vi "Run.vi"(8 "error in (no error)":errorcluster, 11 "Opctics in":refnum<class "Optics.lvclass">) -> (0 "error out":errorcluster, 3 "Optics out":refnum<class "Optics.lvclass">)   [LabVIEW 2018, in "Optics.lvclass"]
uses:
  Optics.lvclass
  C:/Users/observer/Desktop/Sparc4GUI/SPARC4_GUI/Device/Device.lvclass
  Optics.lvclass/Optics.ctl
  Device.lvclass/Device.ctl
  Device.lvclass
  StateMachine/State Machine.lvclass
panel:
  out "on target 2":bool
  out "moving2 2":bool
  out "moving1 2":bool
  out "moving3 2":bool
  out "moving3":bool
  out "moving2":bool
  out "moving1":bool
  out "on target":bool
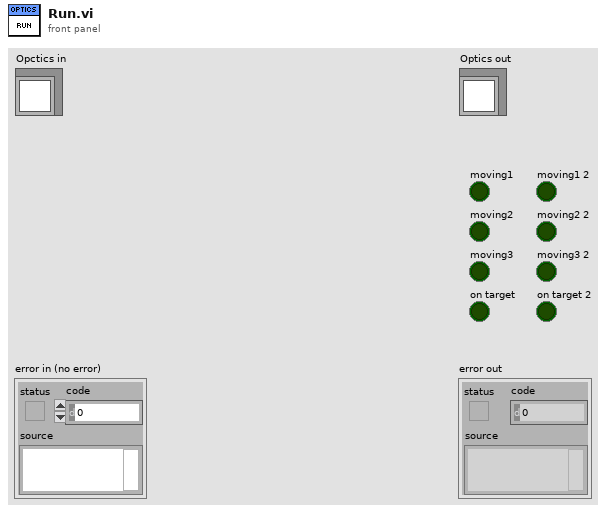
[diagram p1: front panel]
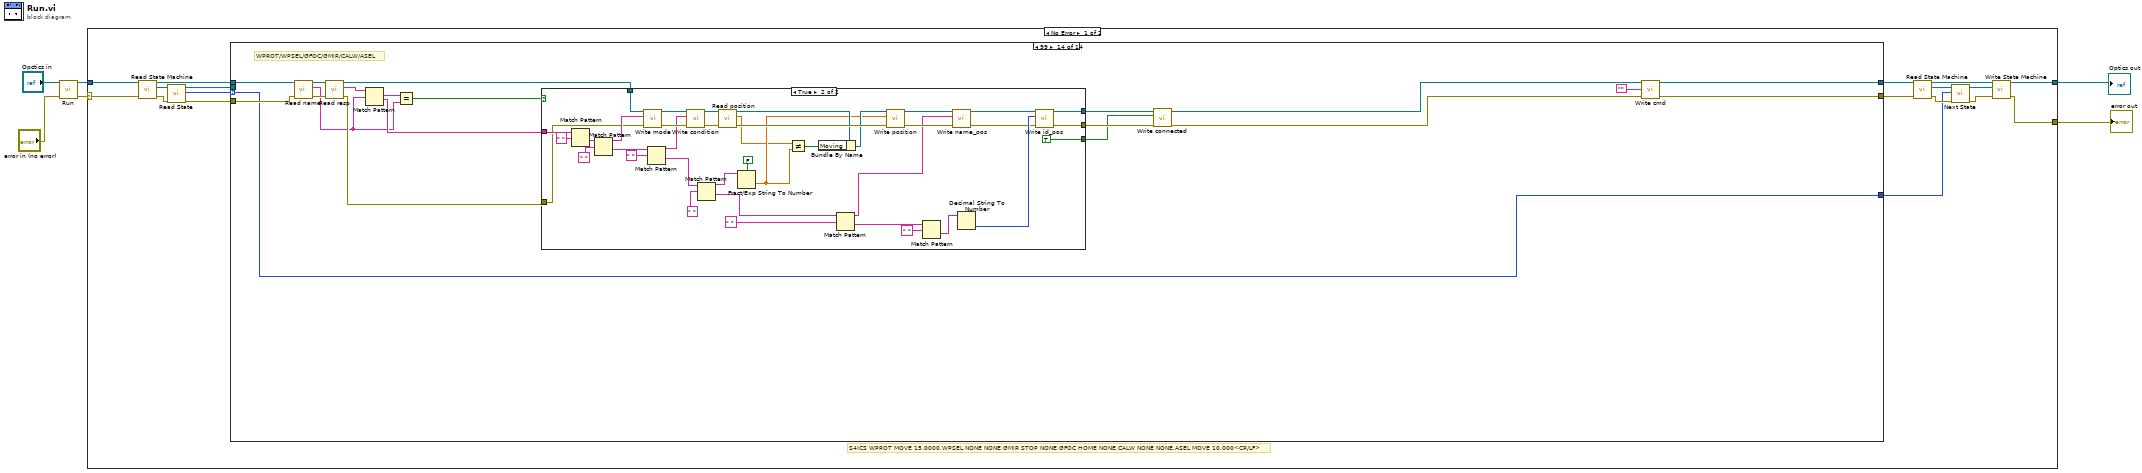
[diagram p0: block diagram]
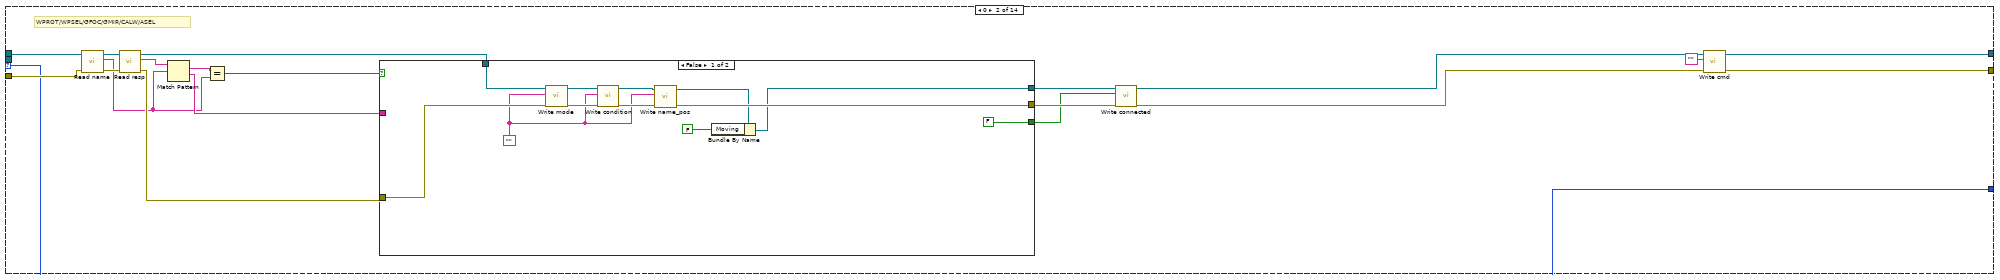
[diagram p3: hidden frame]
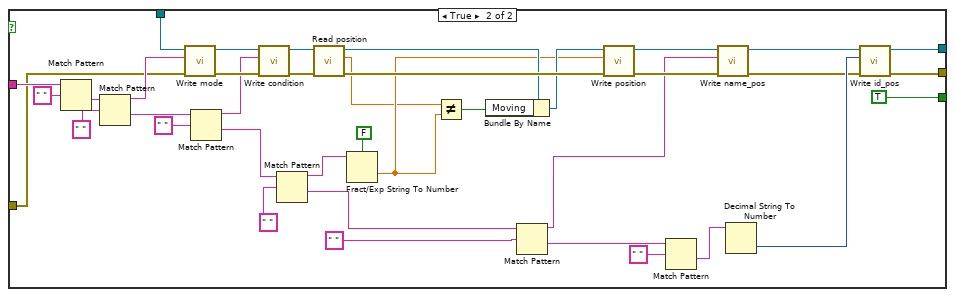
[diagram p4: hidden frame]
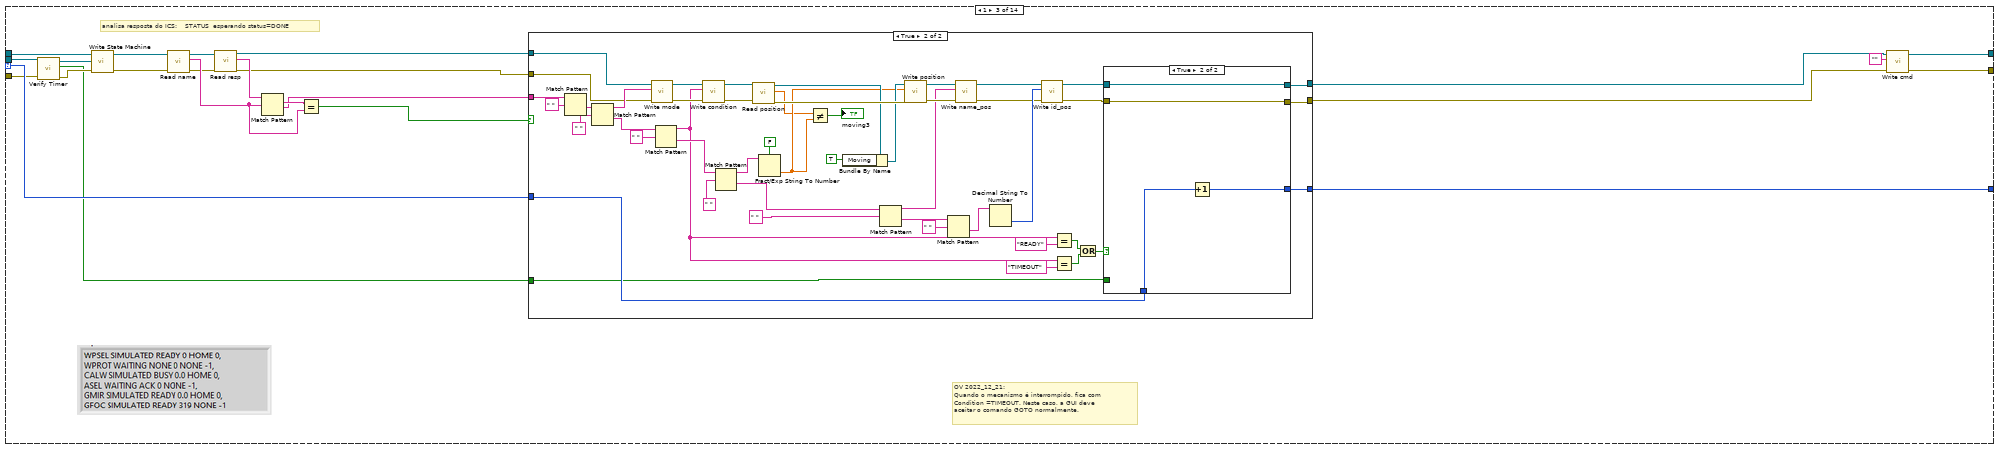
[diagram p5: hidden frame]
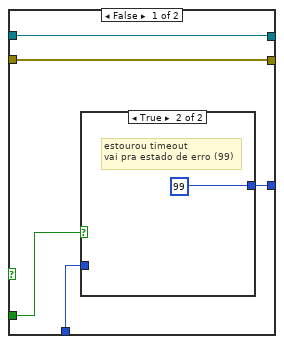
[diagram p7: hidden frame]
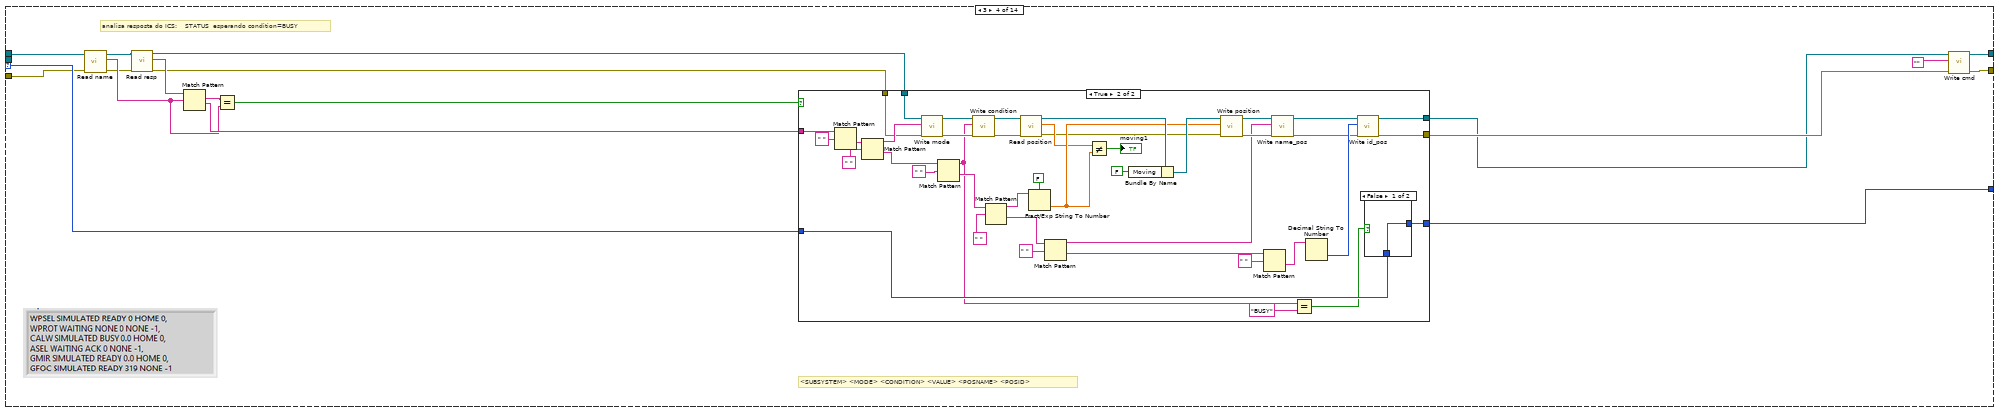
[diagram p9: hidden frame]
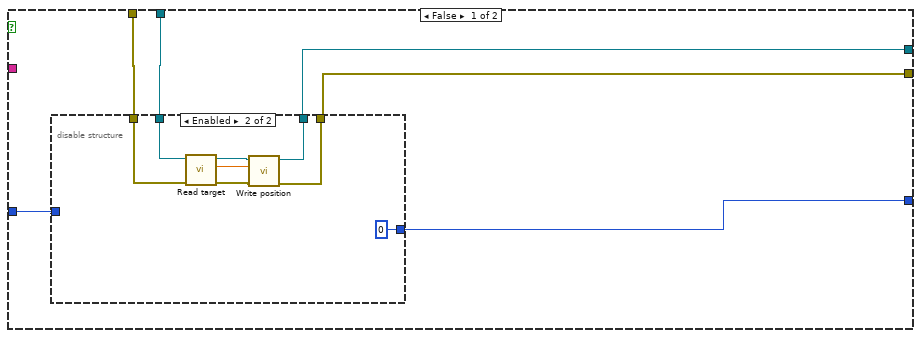
[diagram p10: hidden frame]
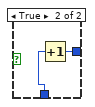
[diagram p12: hidden frame]
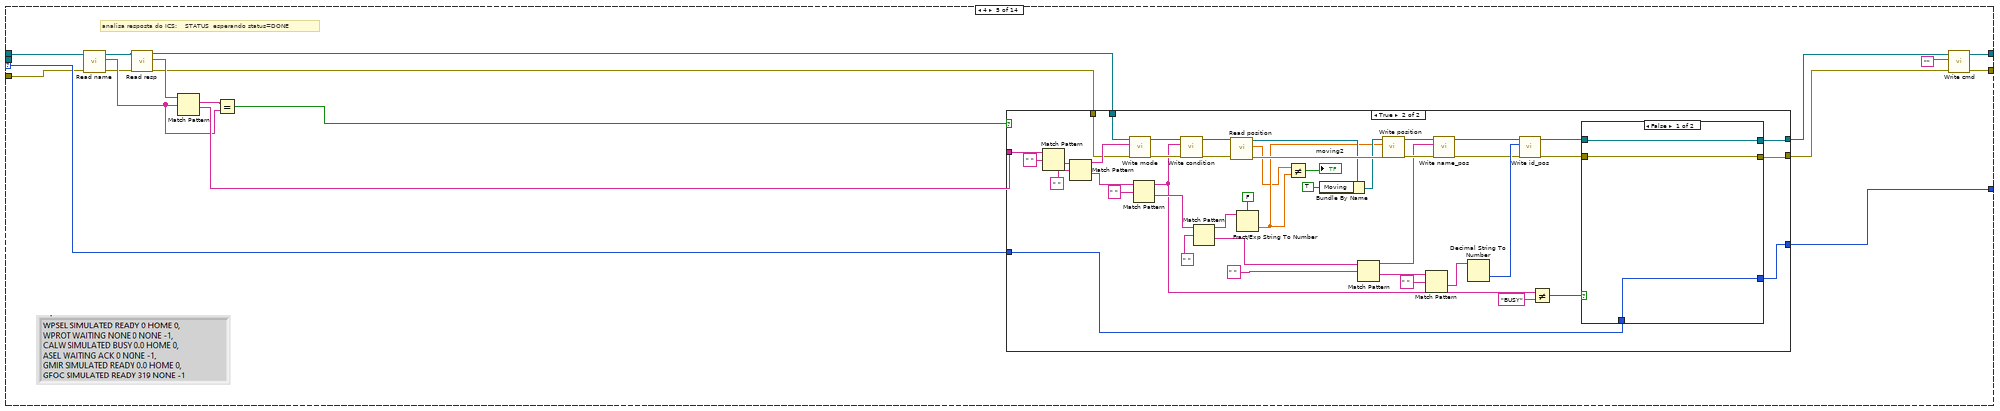
[diagram p13: hidden frame]
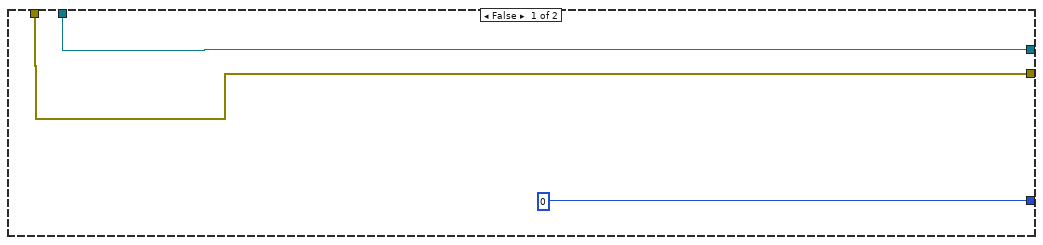
[diagram p14: hidden frame]
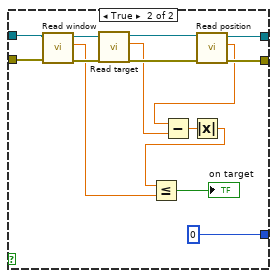
[diagram p15: hidden frame]
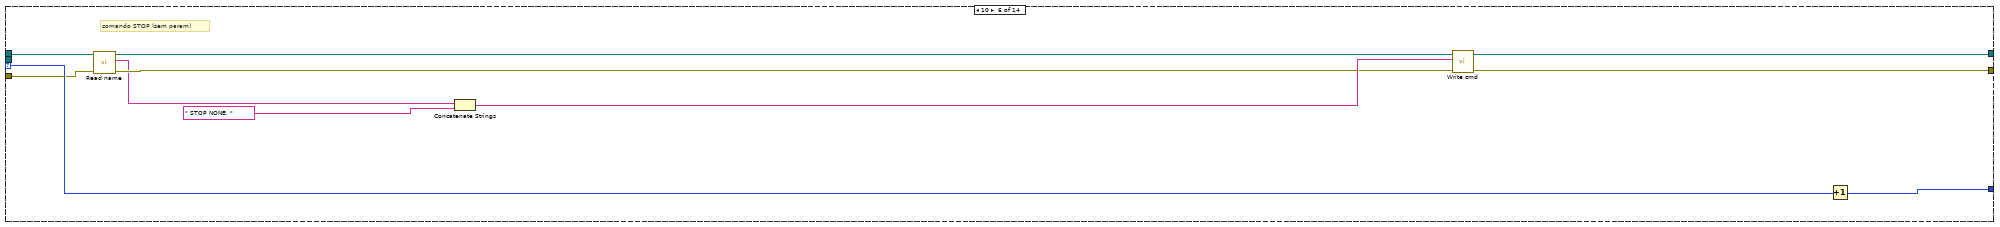
[diagram p16: hidden frame]
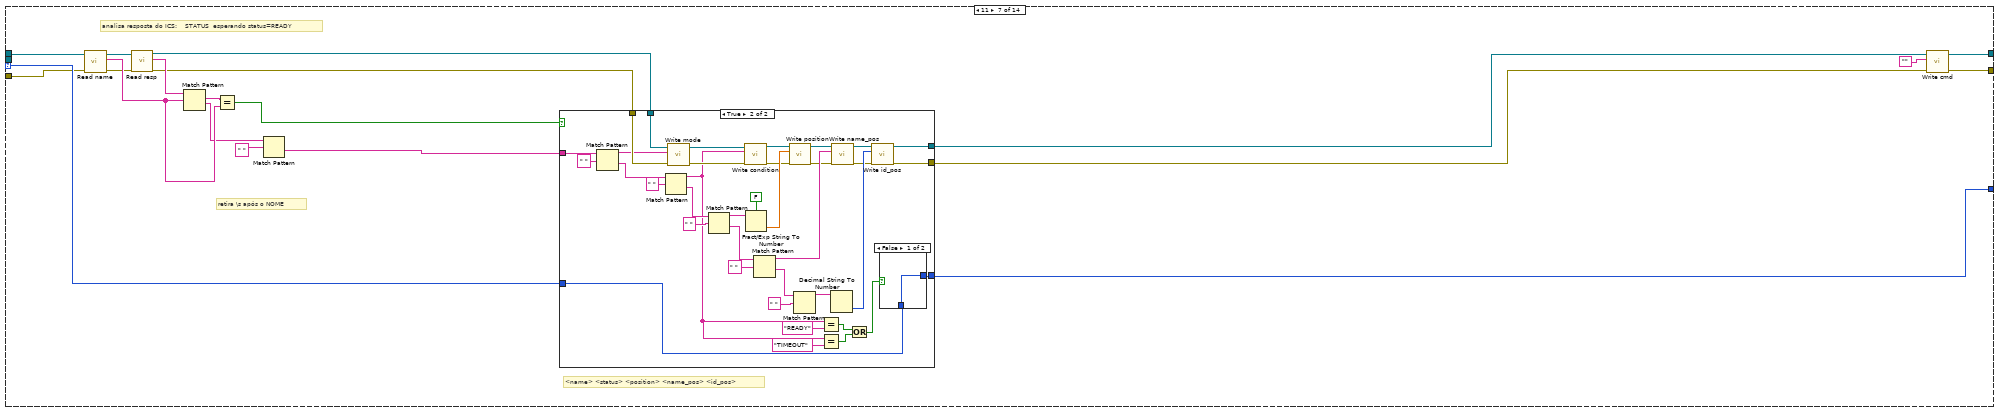
[diagram p17: hidden frame]
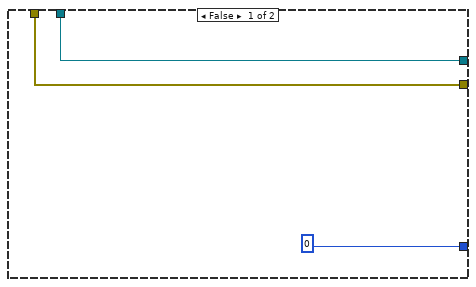
[diagram p18: hidden frame]
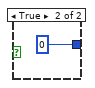
[diagram p19: hidden frame]
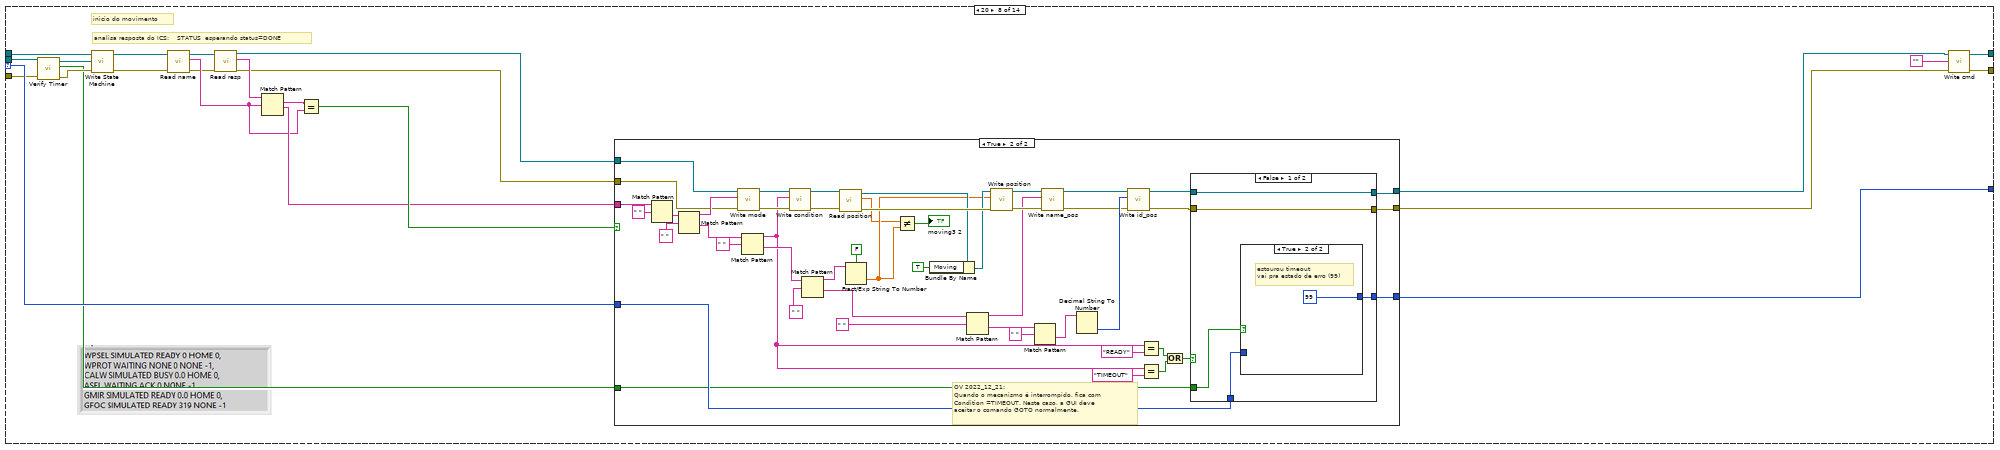
[diagram p20: hidden frame]
diagram:
  n1 = call-parent "Run.vi"("error in (no error)"="error in (no error)", "Device in"="Opctics in") -> ("error out"=w4:errorcluster, "Device out"=w3:refnum<class "Optics.lvclass">)  [unwired: 8 in]
  n2 = case shown="No Error" w4 {
    selector: w4 -> [w7 w884]
    tunnel: [w10 w884] -> w1
    tunnel: [w15 w883] -> w2
    tunnel: w3 -> [w8 w883]
    frame No Error {
      # "S4ICS WPROT MOVE 15.0000,WPSEL NONE NONE,GMIR STOP NONE,GFOC HOME NONE,CALW NONE NONE,ASEL MOVE 10.000<CR/LF>"
      n3 = call-dynamic "Read State Machine.vi"("error in (no error)"=w7, "Device in"=w8) -> ("error out"=w22:errorcluster, "State Machine.lvclass"=w24:refnum<class "State Machine.lvclass">, "Device out"=w20:refnum<class "Optics.lvclass">)  [unwired: 7 in]
      n4 = call-dynamic "Read State.vi"("error in (no error)"=w22, "State Machine in"=w24) -> ("error out"=w21:errorcluster, "State"=w23:i32, "State Machine out"=w9:refnum<class "State Machine.lvclass">)  [unwired: 7 in]
      n5 = case shown="99" w23 {
        selector: w23 -> [w25 w36 w112 w195 w270 w352 w370 w432 w515 w590 w671 w693 w767 w830]
        tunnel: w21 -> [w26 w45 w103 w189 w266 w347 w363 w423 w509 w586 w668 w683 w754 w839]
        tunnel: [w26 w46 w118 w192 w276 w354 w367 w438 w512 w596 w674 w690 w764 w840] -> w11
        tunnel: w20 -> [w27 w44 w108 w191 w269 w349 w366 w428 w511 w589 w669 w686 w757 w838]
        tunnel: [w27 w47 w119 w193 w277 w355 w368 w439 w513 w597 w675 w691 w765 w841] -> w18
        tunnel: [w25 w36 w113 w194 w271 w353 w369 w433 w514 w591 w672 w692 w766 w830] -> w12
        tunnel: w9 -> [_ _ w107 _ _ _ _ w427 _ _ _ w684 w756 _]
        frame Default {
        }
        frame 0 {
          # "WPROT/WPSEL/GFOC/GMIR/CALW/ASEL"
          n6 = call "Read name.vi"("error in (no error)"=w45, "Optics in"=w44) -> ("error out"=w39:errorcluster, "name"=w34:string, "Optics out"=w41:refnum<class "Optics.lvclass">)  [unwired: 7 in]
          n7 = call-dynamic "Read resp.vi"("error in (no error)"=w39, "Device in"=w41) -> ("error out"=w38:errorcluster, "resp"=w43:string, "Device out"=w40:refnum<class "Optics.lvclass">)  [unwired: 7 in]
          n8 = Match Pattern(string=w43, regular expression=w34) -> (match substring=w42:string, after substring=w35:string)  [unwired: 1 in, 2 out]
          n9 = Equal?(x=w42, y=w34) -> (x = y?=w37:bool)
          n10 = case shown="False" w37 {
            tunnel: w35 -> [_ w97]
            tunnel: w40 -> [w56 w81]
            tunnel: w38 -> [w55 w71]
            tunnel: [w49 w73] -> w33
            tunnel: [w52 w72] -> w32
            tunnel: [FALSE TRUE] -> w29
            frame False {
              w51 = "" ("string")
              n11 = call "Write mode.vi"("error in (no error)"=w55, "mode"=w51, "Optics in"=w56) -> ("error out"=w58:errorcluster, "Optics out"=w57:refnum<class "Optics.lvclass">)  [unwired: 7 in]
              n12 = call "Write condition.vi"("error in (no error)"=w58, "condition"=w51, "Optics in"=w57) -> ("error out"=w53:errorcluster, "Optics out"=w54:refnum<class "Optics.lvclass">)  [unwired: 7 in]
              n13 = call "Write name_pos.vi"("error in (no error)"=w53, "name_pos"=w51, "Optics in"=w54) -> ("error out"=w52:errorcluster, "Optics out"=w50:refnum<class "Optics.lvclass">)  [unwired: 7 in]
              n14 = Bundle By Name(cluster=w50, "Moving"=FALSE) -> (w49:refnum<class "Optics.lvclass">)
            }
            frame True {
              n15 = Match Pattern(string=w97, regular expression=" ") -> (after substring=w84:string)  [unwired: 1 in, 3 out]
              n16 = Match Pattern(string=w84, regular expression=" ") -> (before substring=w80:string, after substring=w79:string)  [unwired: 1 in, 2 out]
              n17 = call "Write mode.vi"("error in (no error)"=w71, "mode"=w80, "Optics in"=w81) -> ("error out"=w83:errorcluster, "Optics out"=w82:refnum<class "Optics.lvclass">)  [unwired: 7 in]
              n18 = Match Pattern(string=w79, regular expression=" ") -> (before substring=w74:string, after substring=w93:string)  [unwired: 1 in, 2 out]
              n19 = call "Write condition.vi"("error in (no error)"=w83, "condition"=w74, "Optics in"=w82) -> ("error out"=w68:errorcluster, "Optics out"=w69:refnum<class "Optics.lvclass">)  [unwired: 7 in]
              n20 = Match Pattern(string=w93, regular expression=" ") -> (before substring=w78:string, after substring=w90:string)  [unwired: 1 in, 2 out]
              n21 = call "Read position.vi"("error in (no error)"=w68, "Optics in"=w69) -> ("error out"=w67:errorcluster, "position"=w63:dbl, "Optics out"=w66:refnum<class "Optics.lvclass">)  [unwired: 7 in]
              n22 = Fract/Exp String To Number(use system decimal point (T)=FALSE, string=w78) -> (number=w64:dbl)  [unwired: 2 in, 1 out]
              n23 = Not Equal?(x=w63, y=w64) -> (x != y?=w62:bool)
              n24 = Bundle By Name(cluster=w66, "Moving"=w62) -> (w65:refnum<class "Optics.lvclass">)
              n25 = Match Pattern(string=w90, regular expression=" ") -> (before substring=w61:string, after substring=w76:string)  [unwired: 1 in, 2 out]
              n26 = call "Write position.vi"("error in (no error)"=w67, "position"=w64, "Optics in"=w65) -> ("error out"=w87:errorcluster, "Optics out"=w92:refnum<class "Optics.lvclass">)  [unwired: 7 in]
              n27 = Match Pattern(string=w76, regular expression=" ") -> (after substring=w75:string)  [unwired: 1 in, 3 out]
              n28 = call "Write name_pos.vi"("error in (no error)"=w87, "name_pos"=w61, "Optics in"=w92) -> ("error out"=w86:errorcluster, "Optics out"=w88:refnum<class "Optics.lvclass">)  [unwired: 7 in]
              n29 = Decimal String To Number(string=w75) -> (number=w89:i32)  [unwired: 2 in, 1 out]
              n30 = call "Write id_pos.vi"("error in (no error)"=w86, "id_pos"=w89, "Optics in"=w88) -> ("error out"=w72:errorcluster, "Optics out"=w73:refnum<class "Optics.lvclass">)  [unwired: 7 in]
            }
          }
          n31 = call "Write connected.vi"("error in (no error)"=w32, "connected"=w29, "Device in"=w33) -> ("error out"=w30:errorcluster, "Device out"=w31:refnum<class "Optics.lvclass">)  [unwired: 7 in]
          n32 = call-dynamic "Write cmd.vi"("error in (no error)"=w30, "cmd"="", "Device in"=w31) -> ("error out"=w46:errorcluster, "Device out"=w47:refnum<class "Optics.lvclass">)  [unwired: 7 in]
        }
        frame 1 {
          # "OV 2022_12_21:\nQuando o mecanismo é interrompido, fica com\nCondition =TIMEOUT. Neste caso, a GUI deve\naceitar o comando GOTO normalmente."
          # "analisa resposta do ICS:    STATUS  esperando status=DONE"
          n33 = call "Verify Timer.vi"("error in (no error)"=w103, "State Machine in"=w107) -> ("error out"=w102:errorcluster, "timeout"=w101:bool, "State Machine out"=w106:refnum<class "State Machine.lvclass">)  [unwired: 7 in]
          n34 = call-dynamic "Write State Machine.vi"("error in (no error)"=w102, "State Machine.lvclass"=w106, "Device in"=w108) -> ("error out"=w104:errorcluster, "Device out"=w105:refnum<class "Optics.lvclass">)  [unwired: 7 in]
          n35 = call "Read name.vi"("error in (no error)"=w104, "Optics in"=w105) -> ("error out"=w109:errorcluster, "name"=w110:string, "Optics out"=w111:refnum<class "Optics.lvclass">)  [unwired: 7 in]
          n36 = call-dynamic "Read resp.vi"("error in (no error)"=w109, "Device in"=w111) -> ("error out"=w116:errorcluster, "resp"=w121:string, "Device out"=w117:refnum<class "Optics.lvclass">)  [unwired: 7 in]
          n37 = Match Pattern(string=w121, regular expression=w110) -> (match substring=w120:string, after substring=w114:string)  [unwired: 1 in, 2 out]
          n38 = Equal?(x=w120, y=w110) -> (x = y?=w115:bool)
          n39 = case shown="True" w115 {
            tunnel: w114 -> [_ w172]
            tunnel: w117 -> [w123 w156]
            tunnel: w116 -> [w124 w148]
            tunnel: [w123 w142] -> w99
            tunnel: [w124 w141] -> w100
            tunnel: w112 -> [w122 w146]
            tunnel: [w122 w147] -> w113
            tunnel: w101 -> [_ w130]
            frame False {
            }
            frame True {
              n40 = Match Pattern(string=w172, regular expression=" ") -> (after substring=w159:string)  [unwired: 1 in, 3 out]
              n41 = Match Pattern(string=w159, regular expression=" ") -> (before substring=w155:string, after substring=w154:string)  [unwired: 1 in, 2 out]
              n42 = call "Write mode.vi"("error in (no error)"=w148, "mode"=w155, "Optics in"=w156) -> ("error out"=w158:errorcluster, "Optics out"=w157:refnum<class "Optics.lvclass">)  [unwired: 7 in]
              n43 = Match Pattern(string=w154, regular expression=" ") -> (before substring=w128:string, after substring=w168:string)  [unwired: 1 in, 2 out]
              n44 = call "Write condition.vi"("error in (no error)"=w158, "condition"=w128, "Optics in"=w157) -> ("error out"=w138:errorcluster, "Optics out"=w139:refnum<class "Optics.lvclass">)  [unwired: 7 in]
              n45 = Match Pattern(string=w168, regular expression=" ") -> (before substring=w153:string, after substring=w165:string)  [unwired: 1 in, 2 out]
              n46 = call "Read position.vi"("error in (no error)"=w138, "Optics in"=w139) -> ("error out"=w137:errorcluster, "position"=w133:dbl, "Optics out"=w136:refnum<class "Optics.lvclass">)  [unwired: 7 in]
              n47 = Fract/Exp String To Number(use system decimal point (T)=FALSE, string=w153) -> (number=w134:dbl)  [unwired: 2 in, 1 out]
              n48 = Not Equal?(x=w133, y=w134) -> (x != y?=→"moving3":bool)
              n49 = Bundle By Name(cluster=w136, "Moving"=TRUE) -> (w135:refnum<class "Optics.lvclass">)
              n50 = Match Pattern(string=w165, regular expression=" ") -> (before substring=w152:string, after substring=w150:string)  [unwired: 1 in, 2 out]
              n51 = call "Write position.vi"("error in (no error)"=w137, "position"=w134, "Optics in"=w135) -> ("error out"=w162:errorcluster, "Optics out"=w167:refnum<class "Optics.lvclass">)  [unwired: 7 in]
              n52 = Match Pattern(string=w150, regular expression=" ") -> (after substring=w149:string)  [unwired: 1 in, 3 out]
              n53 = call "Write name_pos.vi"("error in (no error)"=w162, "name_pos"=w152, "Optics in"=w167) -> ("error out"=w161:errorcluster, "Optics out"=w163:refnum<class "Optics.lvclass">)  [unwired: 7 in]
              n54 = Decimal String To Number(string=w149) -> (number=w164:i32)  [unwired: 2 in, 1 out]
              n55 = call "Write id_pos.vi"("error in (no error)"=w161, "id_pos"=w164, "Optics in"=w163) -> ("error out"=w143:errorcluster, "Optics out"=w144:refnum<class "Optics.lvclass">)  [unwired: 7 in]
              n56 = Equal?(x=w128, y="READY") -> (x = y?=w126:bool)
              n57 = Equal?(x=w128, y="TIMEOUT") -> (x = y?=w125:bool)
              n58 = Or(x=w126, y=w125) -> (x .or. y?=w127:bool)
              n59 = case shown="True" w127 {
                tunnel: [w175 w180] -> w147
                tunnel: w146 -> [w174 w181]
                tunnel: w144 -> [w177 w183]
                tunnel: w143 -> [w176 w182]
                tunnel: [w177 w183] -> w142
                tunnel: [w176 w182] -> w141
                tunnel: w130 -> [w173 _]
                frame False {
                  n60 = case shown="True" w173 {
                    tunnel: [w178 99 ("State")] -> w175
                    tunnel: w174 -> [w178 _]
                    frame False {
                      # "Não estourou timeout"
                    }
                    frame True {
                      # "estourou timeout\nvai pra estado de erro (99)"
                    }
                  }
                }
                frame True {
                  n61 = Increment(x=w181) -> (x+1=w180:i32)
                }
              }
            }
          }
          n62 = call-dynamic "Write cmd.vi"("error in (no error)"=w100, "cmd"="", "Device in"=w99) -> ("error out"=w118:errorcluster, "Device out"=w119:refnum<class "Optics.lvclass">)  [unwired: 7 in]
        }
        frame 3 {
          # "<SUBSYSTEM> <MODE> <CONDITION> <VALUE> <POSNAME> <POSID>"
          # "analisa resposta do ICS:    STATUS  esperando condition=BUSY"
          n63 = call "Read name.vi"("error in (no error)"=w189, "Optics in"=w191) -> ("error out"=w187:errorcluster, "name"=w188:string, "Optics out"=w190:refnum<class "Optics.lvclass">)  [unwired: 7 in]
          n64 = call-dynamic "Read resp.vi"("error in (no error)"=w187, "Device in"=w190) -> ("error out"=w196:errorcluster, "resp"=w201:string, "Device out"=w197:refnum<class "Optics.lvclass">)  [unwired: 7 in]
          n65 = Match Pattern(string=w201, regular expression=w188) -> (match substring=w199:string, after substring=w198:string)  [unwired: 1 in, 2 out]
          n66 = Equal?(x=w199, y=w188) -> (x = y?=w200:bool)
          n67 = case shown="True" w200 {
            tunnel: w198 -> [_ w258]
            tunnel: w197 -> [w205 w238]
            tunnel: w196 -> [w204 w230]
            tunnel: [w203 w246] -> w184
            tunnel: [w202 w245] -> w185
            tunnel: w195 -> [w207 w243]
            tunnel: [w206 w244] -> w194
            frame False {
              n68 = disable-structure shown="Enabled" {
                disable-tunnel: w207 -> [w208 _]
                disable-tunnel: [w208 0 ("State")] -> w206
                disable-tunnel: w205 -> [_ w216]
                disable-tunnel: w204 -> [_ w215]
                disable-tunnel: [_ w210] -> w203
                disable-tunnel: [_ w209] -> w202
                frame Disabled {
                }
                frame Enabled {
                  n69 = call "Read target.vi"("error in (no error)"=w215, "Optics in"=w216) -> ("error out"=w213:errorcluster, "target"=w212:dbl, "Optics out"=w214:refnum<class "Optics.lvclass">)  [unwired: 7 in]
                  n70 = call "Write position.vi"("error in (no error)"=w213, "position"=w212, "Optics in"=w214) -> ("error out"=w209:errorcluster, "Optics out"=w210:refnum<class "Optics.lvclass">)  [unwired: 7 in]
                }
              }
            }
            frame True {
              n71 = Match Pattern(string=w258, regular expression=" ") -> (after substring=w241:string)  [unwired: 1 in, 3 out]
              n72 = Match Pattern(string=w241, regular expression=" ") -> (before substring=w237:string, after substring=w236:string)  [unwired: 1 in, 2 out]
              n73 = call "Write mode.vi"("error in (no error)"=w230, "mode"=w237, "Optics in"=w238) -> ("error out"=w240:errorcluster, "Optics out"=w239:refnum<class "Optics.lvclass">)  [unwired: 7 in]
              n74 = Match Pattern(string=w236, regular expression=" ") -> (before substring=w220:string, after substring=w254:string)  [unwired: 1 in, 2 out]
              n75 = call "Write condition.vi"("error in (no error)"=w240, "condition"=w220, "Optics in"=w239) -> ("error out"=w228:errorcluster, "Optics out"=w229:refnum<class "Optics.lvclass">)  [unwired: 7 in]
              n76 = Match Pattern(string=w254, regular expression=" ") -> (before substring=w235:string, after substring=w251:string)  [unwired: 1 in, 2 out]
              n77 = call "Read position.vi"("error in (no error)"=w228, "Optics in"=w229) -> ("error out"=w223:errorcluster, "position"=w224:dbl, "Optics out"=w227:refnum<class "Optics.lvclass">)  [unwired: 7 in]
              n78 = Fract/Exp String To Number(use system decimal point (T)=FALSE, string=w235) -> (number=w225:dbl)  [unwired: 2 in, 1 out]
              n79 = Match Pattern(string=w251, regular expression=" ") -> (before substring=w234:string, after substring=w232:string)  [unwired: 1 in, 2 out]
              n80 = Not Equal?(x=w224, y=w225) -> (x != y?=→"moving1":bool)
              n81 = Bundle By Name(cluster=w227, "Moving"=FALSE) -> (w226:refnum<class "Optics.lvclass">)
              n82 = call "Write position.vi"("error in (no error)"=w223, "position"=w225, "Optics in"=w226) -> ("error out"=w248:errorcluster, "Optics out"=w253:refnum<class "Optics.lvclass">)  [unwired: 7 in]
              n83 = Match Pattern(string=w232, regular expression=" ") -> (after substring=w231:string)  [unwired: 1 in, 3 out]
              n84 = call "Write name_pos.vi"("error in (no error)"=w248, "name_pos"=w234, "Optics in"=w253) -> ("error out"=w247:errorcluster, "Optics out"=w249:refnum<class "Optics.lvclass">)  [unwired: 7 in]
              n85 = Equal?(x=w220, y="BUSY") -> (x = y?=w217:bool)
              n86 = Decimal String To Number(string=w231) -> (number=w250:i32)  [unwired: 2 in, 1 out]
              n87 = call "Write id_pos.vi"("error in (no error)"=w247, "id_pos"=w250, "Optics in"=w249) -> ("error out"=w245:errorcluster, "Optics out"=w246:refnum<class "Optics.lvclass">)  [unwired: 7 in]
              n88 = case shown="False" w217 {
                tunnel: [w259 w260] -> w244
                tunnel: w243 -> [w259 w261]
                frame False {
                }
                frame True {
                  n89 = Increment(x=w261) -> (x+1=w260:i32)
                }
              }
            }
          }
          n90 = call-dynamic "Write cmd.vi"("error in (no error)"=w185, "cmd"="", "Device in"=w184) -> ("error out"=w192:errorcluster, "Device out"=w193:refnum<class "Optics.lvclass">)  [unwired: 7 in]
        }
        frame 4 {
          # "analisa resposta do ICS:    STATUS  esperando status=DONE"
          n91 = call "Read name.vi"("error in (no error)"=w266, "Optics in"=w269) -> ("error out"=w265:errorcluster, "name"=w267:string, "Optics out"=w268:refnum<class "Optics.lvclass">)  [unwired: 7 in]
          n92 = call-dynamic "Read resp.vi"("error in (no error)"=w265, "Device in"=w268) -> ("error out"=w274:errorcluster, "resp"=w279:string, "Device out"=w275:refnum<class "Optics.lvclass">)  [unwired: 7 in]
          n93 = Match Pattern(string=w279, regular expression=w267) -> (match substring=w278:string, after substring=w272:string)  [unwired: 1 in, 2 out]
          n94 = Equal?(x=w278, y=w267) -> (x = y?=w273:bool)
          n95 = case shown="True" w273 {
            tunnel: w272 -> [_ w326]
            tunnel: w275 -> [w281 w310]
            tunnel: w274 -> [w282 w302]
            tunnel: [w281 w294] -> w263
            tunnel: [w282 w293] -> w264
            tunnel: w270 -> [_ w300]
            tunnel: [0 w301] -> w271
            frame False {
            }
            frame True {
              n96 = Match Pattern(string=w326, regular expression=" ") -> (after substring=w313:string)  [unwired: 1 in, 3 out]
              n97 = Match Pattern(string=w313, regular expression=" ") -> (before substring=w309:string, after substring=w308:string)  [unwired: 1 in, 2 out]
              n98 = call "Write mode.vi"("error in (no error)"=w302, "mode"=w309, "Optics in"=w310) -> ("error out"=w312:errorcluster, "Optics out"=w311:refnum<class "Optics.lvclass">)  [unwired: 7 in]
              n99 = Match Pattern(string=w308, regular expression=" ") -> (before substring=w297:string, after substring=w322:string)  [unwired: 1 in, 2 out]
              n100 = call "Write condition.vi"("error in (no error)"=w312, "condition"=w297, "Optics in"=w311) -> ("error out"=w290:errorcluster, "Optics out"=w291:refnum<class "Optics.lvclass">)  [unwired: 7 in]
              n101 = Match Pattern(string=w322, regular expression=" ") -> (before substring=w307:string, after substring=w319:string)  [unwired: 1 in, 2 out]
              n102 = call "Read position.vi"("error in (no error)"=w290, "Optics in"=w291) -> ("error out"=w289:errorcluster, "position"=w285:dbl, "Optics out"=w288:refnum<class "Optics.lvclass">)  [unwired: 7 in]
              n103 = Fract/Exp String To Number(use system decimal point (T)=FALSE, string=w307) -> (number=w286:dbl)  [unwired: 2 in, 1 out]
              n104 = Not Equal?(x=w285, y=w286) -> (x != y?=→"moving2":bool)
              n105 = Bundle By Name(cluster=w288, "Moving"=TRUE) -> (w287:refnum<class "Optics.lvclass">)
              n106 = Match Pattern(string=w319, regular expression=" ") -> (before substring=w306:string, after substring=w304:string)  [unwired: 1 in, 2 out]
              n107 = call "Write position.vi"("error in (no error)"=w289, "position"=w286, "Optics in"=w287) -> ("error out"=w316:errorcluster, "Optics out"=w321:refnum<class "Optics.lvclass">)  [unwired: 7 in]
              n108 = Match Pattern(string=w304, regular expression=" ") -> (after substring=w303:string)  [unwired: 1 in, 3 out]
              n109 = call "Write name_pos.vi"("error in (no error)"=w316, "name_pos"=w306, "Optics in"=w321) -> ("error out"=w315:errorcluster, "Optics out"=w317:refnum<class "Optics.lvclass">)  [unwired: 7 in]
              n110 = Decimal String To Number(string=w303) -> (number=w318:i32)  [unwired: 2 in, 1 out]
              n111 = call "Write id_pos.vi"("error in (no error)"=w315, "id_pos"=w318, "Optics in"=w317) -> ("error out"=w295:errorcluster, "Optics out"=w296:refnum<class "Optics.lvclass">)  [unwired: 7 in]
              n112 = Not Equal?(x=w297, y="BUSY") -> (x != y?=w298:bool)
              n113 = case shown="False" w298 {
                tunnel: [w329 0 ("t")] -> w301
                tunnel: w300 -> [w329 _]
                tunnel: w296 -> [w328 w336]
                tunnel: w295 -> [w327 w334]
                tunnel: [w328 w342] -> w294
                tunnel: [w327 w341] -> w293
                frame False {
                }
                frame True {
                  n114 = call "Read window.vi"("error in (no error)"=w334, "Optics in"=w336) -> ("error out"=w333:errorcluster, "window"=w332:dbl, "Optics out"=w335:refnum<class "Optics.lvclass">)  [unwired: 7 in]
                  n115 = call "Read target.vi"("error in (no error)"=w333, "Optics in"=w335) -> ("error out"=w344:errorcluster, "target"=w340:dbl, "Optics out"=w343:refnum<class "Optics.lvclass">)  [unwired: 7 in]
                  n116 = call "Read position.vi"("error in (no error)"=w344, "Optics in"=w343) -> ("error out"=w341:errorcluster, "position"=w339:dbl, "Optics out"=w342:refnum<class "Optics.lvclass">)  [unwired: 7 in]
                  n117 = Subtract(x=w339, y=w340) -> (x-y=w338:dbl)
                  n118 = Absolute Value(x=w338) -> (abs(x)=w337:dbl)
                  n119 = Less Or Equal?(x=w337, y=w332) -> (x <= y?=→"on target":bool)
                }
              }
            }
          }
          n120 = call-dynamic "Write cmd.vi"("error in (no error)"=w264, "cmd"="", "Device in"=w263) -> ("error out"=w276:errorcluster, "Device out"=w277:refnum<class "Optics.lvclass">)  [unwired: 7 in]
        }
        frame 10 {
          # "comando STOP (sem param)"
          n121 = call "Read name.vi"("error in (no error)"=w347, "Optics in"=w349) -> ("error out"=w346:errorcluster, "name"=w345:string, "Optics out"=w348:refnum<class "Optics.lvclass">)  [unwired: 7 in]
          n122 = Concatenate Strings(w345, " STOP NONE, " ("string")) -> (w350:string)
          n123 = call-dynamic "Write cmd.vi"("error in (no error)"=w346, "cmd"=w350, "Device in"=w348) -> ("error out"=w354:errorcluster, "Device out"=w355:refnum<class "Optics.lvclass">)  [unwired: 7 in]
          n124 = Increment(x=w352) -> (x+1=w353:i32)
        }
        frame 11 {
          # "retira \\s após o NOME"
          # "<name> <status> <position> <name_pos> <id_pos>"
          # "analisa resposta do ICS:    STATUS  esperando status=READY"
          n125 = call "Read name.vi"("error in (no error)"=w363, "Optics in"=w366) -> ("error out"=w362:errorcluster, "name"=w364:string, "Optics out"=w365:refnum<class "Optics.lvclass">)  [unwired: 7 in]
          n126 = call-dynamic "Read resp.vi"("error in (no error)"=w362, "Device in"=w365) -> ("error out"=w371:errorcluster, "resp"=w375:string, "Device out"=w372:refnum<class "Optics.lvclass">)  [unwired: 7 in]
          n127 = Match Pattern(string=w375, regular expression=w364) -> (match substring=w373:string, after substring=w361:string)  [unwired: 1 in, 2 out]
          n128 = Equal?(x=w373, y=w364) -> (x = y?=w374:bool)
          n129 = Match Pattern(string=w361, regular expression=" ") -> (after substring=w360:string)  [unwired: 1 in, 3 out]
          n130 = case shown="True" w374 {
            tunnel: w360 -> [_ w391]
            tunnel: w372 -> [w378 w389]
            tunnel: w371 -> [w377 w388]
            tunnel: [w378 w397] -> w357
            tunnel: [w377 w396] -> w356
            tunnel: w370 -> [_ w393]
            tunnel: [0 ("State") w395] -> w369
            frame False {
            }
            frame True {
              n131 = Match Pattern(string=w391, regular expression=" ") -> (before substring=w387:string, after substring=w390:string)  [unwired: 1 in, 2 out]
              n132 = Match Pattern(string=w390, regular expression=" ") -> (before substring=w379:string, after substring=w413:string)  [unwired: 1 in, 2 out]
              n133 = call "Write mode.vi"("error in (no error)"=w388, "mode"=w387, "Optics in"=w389) -> ("error out"=w385:errorcluster, "Optics out"=w386:refnum<class "Optics.lvclass">)  [unwired: 7 in]
              n134 = Match Pattern(string=w413, regular expression=" ") -> (before substring=w409:string, after substring=w408:string)  [unwired: 1 in, 2 out]
              n135 = call "Write condition.vi"("error in (no error)"=w385, "condition"=w379, "Optics in"=w386) -> ("error out"=w400:errorcluster, "Optics out"=w412:refnum<class "Optics.lvclass">)  [unwired: 7 in]
              n136 = Fract/Exp String To Number(use system decimal point (T)=FALSE, string=w409) -> (number=w410:dbl)  [unwired: 2 in, 1 out]
              n137 = Match Pattern(string=w408, regular expression=" ") -> (before substring=w407:string, after substring=w404:string)  [unwired: 1 in, 2 out]
              n138 = call "Write position.vi"("error in (no error)"=w400, "position"=w410, "Optics in"=w412) -> ("error out"=w399:errorcluster, "Optics out"=w406:refnum<class "Optics.lvclass">)  [unwired: 7 in]
              n139 = Match Pattern(string=w404, regular expression=" ") -> (before substring=w403:string)  [unwired: 1 in, 3 out]
              n140 = Equal?(x=w379, y="TIMEOUT") -> (x = y?=w381:bool)
              n141 = Equal?(x=w379, y="READY") -> (x = y?=w382:bool)
              n142 = Decimal String To Number(string=w403) -> (number=w402:i32)  [unwired: 2 in, 1 out]
              n143 = call "Write name_pos.vi"("error in (no error)"=w399, "name_pos"=w407, "Optics in"=w406) -> ("error out"=w398:errorcluster, "Optics out"=w401:refnum<class "Optics.lvclass">)  [unwired: 7 in]
              n144 = Or(x=w382, y=w381) -> (x .or. y?=w380:bool)
              n145 = call "Write id_pos.vi"("error in (no error)"=w398, "id_pos"=w402, "Optics in"=w401) -> ("error out"=w396:errorcluster, "Optics out"=w397:refnum<class "Optics.lvclass">)  [unwired: 7 in]
              n146 = case shown="False" w380 {
                tunnel: [w416 0] -> w395
                tunnel: w393 -> [w416 _]
                frame False {
                }
                frame True {
                }
              }
            }
          }
          n147 = call-dynamic "Write cmd.vi"("error in (no error)"=w356, "cmd"="", "Device in"=w357) -> ("error out"=w367:errorcluster, "Device out"=w368:refnum<class "Optics.lvclass">)  [unwired: 7 in]
        }
        frame 20 {
          # "inicio do movimento"
          # "OV 2022_12_21:\nQuando o mecanismo é interrompido, fica com\nCondition =TIMEOUT. Neste caso, a GUI deve\naceitar o comando GOTO normalmente."
          # "analisa resposta do ICS:    STATUS  esperando status=DONE"
          n148 = call "Verify Timer.vi"("error in (no error)"=w423, "State Machine in"=w427) -> ("error out"=w422:errorcluster, "timeout"=w421:bool, "State Machine out"=w426:refnum<class "State Machine.lvclass">)  [unwired: 7 in]
          n149 = call-dynamic "Write State Machine.vi"("error in (no error)"=w422, "State Machine.lvclass"=w426, "Device in"=w428) -> ("error out"=w424:errorcluster, "Device out"=w425:refnum<class "Optics.lvclass">)  [unwired: 7 in]
          n150 = call "Read name.vi"("error in (no error)"=w424, "Optics in"=w425) -> ("error out"=w429:errorcluster, "name"=w430:string, "Optics out"=w431:refnum<class "Optics.lvclass">)  [unwired: 7 in]
          n151 = call-dynamic "Read resp.vi"("error in (no error)"=w429, "Device in"=w431) -> ("error out"=w436:errorcluster, "resp"=w441:string, "Device out"=w437:refnum<class "Optics.lvclass">)  [unwired: 7 in]
          n152 = Match Pattern(string=w441, regular expression=w430) -> (match substring=w440:string, after substring=w434:string)  [unwired: 1 in, 2 out]
          n153 = Equal?(x=w440, y=w430) -> (x = y?=w435:bool)
          n154 = case shown="True" w435 {
            tunnel: w434 -> [_ w492]
            tunnel: w437 -> [w443 w476]
            tunnel: w436 -> [w444 w468]
            tunnel: [w443 w462] -> w418
            tunnel: [w444 w461] -> w419
            tunnel: w432 -> [_ w466]
            tunnel: [0 w467] -> w433
            tunnel: w421 -> [_ w450]
            frame False {
            }
            frame True {
              n155 = Match Pattern(string=w492, regular expression=" ") -> (after substring=w479:string)  [unwired: 1 in, 3 out]
              n156 = Match Pattern(string=w479, regular expression=" ") -> (before substring=w475:string, after substring=w474:string)  [unwired: 1 in, 2 out]
              n157 = call "Write mode.vi"("error in (no error)"=w468, "mode"=w475, "Optics in"=w476) -> ("error out"=w478:errorcluster, "Optics out"=w477:refnum<class "Optics.lvclass">)  [unwired: 7 in]
              n158 = Match Pattern(string=w474, regular expression=" ") -> (before substring=w448:string, after substring=w488:string)  [unwired: 1 in, 2 out]
              n159 = call "Write condition.vi"("error in (no error)"=w478, "condition"=w448, "Optics in"=w477) -> ("error out"=w458:errorcluster, "Optics out"=w459:refnum<class "Optics.lvclass">)  [unwired: 7 in]
              n160 = Match Pattern(string=w488, regular expression=" ") -> (before substring=w473:string, after substring=w485:string)  [unwired: 1 in, 2 out]
              n161 = call "Read position.vi"("error in (no error)"=w458, "Optics in"=w459) -> ("error out"=w457:errorcluster, "position"=w453:dbl, "Optics out"=w456:refnum<class "Optics.lvclass">)  [unwired: 7 in]
              n162 = Fract/Exp String To Number(use system decimal point (T)=FALSE, string=w473) -> (number=w454:dbl)  [unwired: 2 in, 1 out]
              n163 = Not Equal?(x=w453, y=w454) -> (x != y?=→"moving3 2":bool)
              n164 = Bundle By Name(cluster=w456, "Moving"=TRUE) -> (w455:refnum<class "Optics.lvclass">)
              n165 = Match Pattern(string=w485, regular expression=" ") -> (before substring=w472:string, after substring=w470:string)  [unwired: 1 in, 2 out]
              n166 = call "Write position.vi"("error in (no error)"=w457, "position"=w454, "Optics in"=w455) -> ("error out"=w482:errorcluster, "Optics out"=w487:refnum<class "Optics.lvclass">)  [unwired: 7 in]
              n167 = Match Pattern(string=w470, regular expression=" ") -> (after substring=w469:string)  [unwired: 1 in, 3 out]
              n168 = call "Write name_pos.vi"("error in (no error)"=w482, "name_pos"=w472, "Optics in"=w487) -> ("error out"=w481:errorcluster, "Optics out"=w483:refnum<class "Optics.lvclass">)  [unwired: 7 in]
              n169 = Decimal String To Number(string=w469) -> (number=w484:i32)  [unwired: 2 in, 1 out]
              n170 = call "Write id_pos.vi"("error in (no error)"=w481, "id_pos"=w484, "Optics in"=w483) -> ("error out"=w463:errorcluster, "Optics out"=w464:refnum<class "Optics.lvclass">)  [unwired: 7 in]
              n171 = Equal?(x=w448, y="READY") -> (x = y?=w446:bool)
              n172 = Equal?(x=w448, y="TIMEOUT") -> (x = y?=w445:bool)
              n173 = Or(x=w446, y=w445) -> (x .or. y?=w447:bool)
              n174 = case shown="False" w447 {
                tunnel: [w495 w500] -> w467
                tunnel: w466 -> [w494 w501]
                tunnel: w464 -> [w497 w503]
                tunnel: w463 -> [w496 w502]
                tunnel: [w497 w503] -> w462
                tunnel: [w496 w502] -> w461
                tunnel: w450 -> [w493 _]
                frame False {
                  n175 = case shown="True" w493 {
                    tunnel: [w498 99 ("State")] -> w495
                    tunnel: w494 -> [w498 _]
                    frame False {
                      # "Não estourou timeout"
                    }
                    frame True {
                      # "estourou timeout\nvai pra estado de erro (99)"
                    }
                  }
                }
                frame True {
                  n176 = Increment(x=w501) -> (x+1=w500:i32)
                }
              }
            }
          }
          n177 = call-dynamic "Write cmd.vi"("error in (no error)"=w419, "cmd"="", "Device in"=w418) -> ("error out"=w438:errorcluster, "Device out"=w439:refnum<class "Optics.lvclass">)  [unwired: 7 in]
        }
        frame 22 {
          # "<SUBSYSTEM> <MODE> <CONDITION> <VALUE> <POSNAME> <POSID>"
          # "analisa resposta do ICS:    STATUS  esperando condition=BUSY"
          n178 = call "Read name.vi"("error in (no error)"=w509, "Optics in"=w511) -> ("error out"=w507:errorcluster, "name"=w508:string, "Optics out"=w510:refnum<class "Optics.lvclass">)  [unwired: 7 in]
          n179 = call-dynamic "Read resp.vi"("error in (no error)"=w507, "Device in"=w510) -> ("error out"=w516:errorcluster, "resp"=w521:string, "Device out"=w517:refnum<class "Optics.lvclass">)  [unwired: 7 in]
          n180 = Match Pattern(string=w521, regular expression=w508) -> (match substring=w519:string, after substring=w518:string)  [unwired: 1 in, 2 out]
          n181 = Equal?(x=w519, y=w508) -> (x = y?=w520:bool)
          n182 = case shown="False" w520 {
            tunnel: w518 -> [_ w578]
            tunnel: w517 -> [w525 w558]
            tunnel: w516 -> [w524 w550]
            tunnel: [w523 w566] -> w505
            tunnel: [w522 w565] -> w506
            tunnel: w515 -> [w527 w563]
            tunnel: [w526 w564] -> w514
            frame False {
              n183 = disable-structure shown="Enabled" {
                disable-tunnel: w527 -> [w528 _]
                disable-tunnel: [w528 0 ("State")] -> w526
                disable-tunnel: w525 -> [_ w536]
                disable-tunnel: w524 -> [_ w535]
                disable-tunnel: [_ w530] -> w523
                disable-tunnel: [_ w529] -> w522
                frame Disabled {
                }
                frame Enabled {
                  n184 = call "Read target.vi"("error in (no error)"=w535, "Optics in"=w536) -> ("error out"=w533:errorcluster, "target"=w532:dbl, "Optics out"=w534:refnum<class "Optics.lvclass">)  [unwired: 7 in]
                  n185 = call "Write position.vi"("error in (no error)"=w533, "position"=w532, "Optics in"=w534) -> ("error out"=w529:errorcluster, "Optics out"=w530:refnum<class "Optics.lvclass">)  [unwired: 7 in]
                }
              }
            }
            frame True {
              n186 = Match Pattern(string=w578, regular expression=" ") -> (after substring=w561:string)  [unwired: 1 in, 3 out]
              n187 = Match Pattern(string=w561, regular expression=" ") -> (before substring=w557:string, after substring=w556:string)  [unwired: 1 in, 2 out]
              n188 = call "Write mode.vi"("error in (no error)"=w550, "mode"=w557, "Optics in"=w558) -> ("error out"=w560:errorcluster, "Optics out"=w559:refnum<class "Optics.lvclass">)  [unwired: 7 in]
              n189 = Match Pattern(string=w556, regular expression=" ") -> (before substring=w540:string, after substring=w574:string)  [unwired: 1 in, 2 out]
              n190 = call "Write condition.vi"("error in (no error)"=w560, "condition"=w540, "Optics in"=w559) -> ("error out"=w548:errorcluster, "Optics out"=w549:refnum<class "Optics.lvclass">)  [unwired: 7 in]
              n191 = Match Pattern(string=w574, regular expression=" ") -> (before substring=w555:string, after substring=w571:string)  [unwired: 1 in, 2 out]
              n192 = call "Read position.vi"("error in (no error)"=w548, "Optics in"=w549) -> ("error out"=w543:errorcluster, "position"=w544:dbl, "Optics out"=w547:refnum<class "Optics.lvclass">)  [unwired: 7 in]
              n193 = Fract/Exp String To Number(use system decimal point (T)=FALSE, string=w555) -> (number=w545:dbl)  [unwired: 2 in, 1 out]
              n194 = Match Pattern(string=w571, regular expression=" ") -> (before substring=w554:string, after substring=w552:string)  [unwired: 1 in, 2 out]
              n195 = Not Equal?(x=w544, y=w545) -> (x != y?=→"moving1 2":bool)
              n196 = Bundle By Name(cluster=w547, "Moving"=FALSE) -> (w546:refnum<class "Optics.lvclass">)
              n197 = call "Write position.vi"("error in (no error)"=w543, "position"=w545, "Optics in"=w546) -> ("error out"=w568:errorcluster, "Optics out"=w573:refnum<class "Optics.lvclass">)  [unwired: 7 in]
              n198 = Match Pattern(string=w552, regular expression=" ") -> (after substring=w551:string)  [unwired: 1 in, 3 out]
              n199 = call "Write name_pos.vi"("error in (no error)"=w568, "name_pos"=w554, "Optics in"=w573) -> ("error out"=w567:errorcluster, "Optics out"=w569:refnum<class "Optics.lvclass">)  [unwired: 7 in]
              n200 = Equal?(x=w540, y="BUSY") -> (x = y?=w537:bool)
              n201 = Decimal String To Number(string=w551) -> (number=w570:i32)  [unwired: 2 in, 1 out]
              n202 = call "Write id_pos.vi"("error in (no error)"=w567, "id_pos"=w570, "Optics in"=w569) -> ("error out"=w565:errorcluster, "Optics out"=w566:refnum<class "Optics.lvclass">)  [unwired: 7 in]
              n203 = case shown="True" w537 {
                tunnel: [w579 w580] -> w564
                tunnel: w563 -> [w579 w581]
                frame False {
                }
                frame True {
                  n204 = Increment(x=w581) -> (x+1=w580:i32)
                }
              }
            }
          }
          n205 = call-dynamic "Write cmd.vi"("error in (no error)"=w506, "cmd"="", "Device in"=w505) -> ("error out"=w512:errorcluster, "Device out"=w513:refnum<class "Optics.lvclass">)  [unwired: 7 in]
        }
        frame 23 {
          # "analisa resposta do ICS:    STATUS  esperando status=DONE"
          n206 = call "Read name.vi"("error in (no error)"=w586, "Optics in"=w589) -> ("error out"=w585:errorcluster, "name"=w587:string, "Optics out"=w588:refnum<class "Optics.lvclass">)  [unwired: 7 in]
          n207 = call-dynamic "Read resp.vi"("error in (no error)"=w585, "Device in"=w588) -> ("error out"=w594:errorcluster, "resp"=w599:string, "Device out"=w595:refnum<class "Optics.lvclass">)  [unwired: 7 in]
          n208 = Match Pattern(string=w599, regular expression=w587) -> (match substring=w598:string, after substring=w592:string)  [unwired: 1 in, 2 out]
          n209 = Equal?(x=w598, y=w587) -> (x = y?=w593:bool)
          n210 = case shown="True" w593 {
            tunnel: w592 -> [_ w646]
            tunnel: w595 -> [w601 w630]
            tunnel: w594 -> [w602 w622]
            tunnel: [w601 w614] -> w583
            tunnel: [w602 w613] -> w582
            tunnel: w590 -> [_ w620]
            tunnel: [0 w621] -> w591
            frame False {
            }
            frame True {
              n211 = Match Pattern(string=w646, regular expression=" ") -> (after substring=w633:string)  [unwired: 1 in, 3 out]
              n212 = Match Pattern(string=w633, regular expression=" ") -> (before substring=w629:string, after substring=w628:string)  [unwired: 1 in, 2 out]
              n213 = call "Write mode.vi"("error in (no error)"=w622, "mode"=w629, "Optics in"=w630) -> ("error out"=w632:errorcluster, "Optics out"=w631:refnum<class "Optics.lvclass">)  [unwired: 7 in]
              n214 = Match Pattern(string=w628, regular expression=" ") -> (before substring=w617:string, after substring=w642:string)  [unwired: 1 in, 2 out]
              n215 = call "Write condition.vi"("error in (no error)"=w632, "condition"=w617, "Optics in"=w631) -> ("error out"=w610:errorcluster, "Optics out"=w611:refnum<class "Optics.lvclass">)  [unwired: 7 in]
              n216 = Match Pattern(string=w642, regular expression=" ") -> (before substring=w627:string, after substring=w639:string)  [unwired: 1 in, 2 out]
              n217 = call "Read position.vi"("error in (no error)"=w610, "Optics in"=w611) -> ("error out"=w609:errorcluster, "position"=w605:dbl, "Optics out"=w608:refnum<class "Optics.lvclass">)  [unwired: 7 in]
              n218 = Fract/Exp String To Number(use system decimal point (T)=FALSE, string=w627) -> (number=w606:dbl)  [unwired: 2 in, 1 out]
              n219 = Not Equal?(x=w605, y=w606) -> (x != y?=→"moving2 2":bool)
              n220 = Bundle By Name(cluster=w608, "Moving"=TRUE) -> (w607:refnum<class "Optics.lvclass">)
              n221 = Match Pattern(string=w639, regular expression=" ") -> (before substring=w626:string, after substring=w624:string)  [unwired: 1 in, 2 out]
              n222 = call "Write position.vi"("error in (no error)"=w609, "position"=w606, "Optics in"=w607) -> ("error out"=w636:errorcluster, "Optics out"=w641:refnum<class "Optics.lvclass">)  [unwired: 7 in]
              n223 = Match Pattern(string=w624, regular expression=" ") -> (after substring=w623:string)  [unwired: 1 in, 3 out]
              n224 = call "Write name_pos.vi"("error in (no error)"=w636, "name_pos"=w626, "Optics in"=w641) -> ("error out"=w635:errorcluster, "Optics out"=w637:refnum<class "Optics.lvclass">)  [unwired: 7 in]
              n225 = Decimal String To Number(string=w623) -> (number=w638:i32)  [unwired: 2 in, 1 out]
              n226 = call "Write id_pos.vi"("error in (no error)"=w635, "id_pos"=w638, "Optics in"=w637) -> ("error out"=w615:errorcluster, "Optics out"=w616:refnum<class "Optics.lvclass">)  [unwired: 7 in]
              n227 = Not Equal?(x=w617, y="BUSY") -> (x != y?=w618:bool)
              n228 = case shown="False" w618 {
                tunnel: [w649 21 ("t")] -> w621
                tunnel: w620 -> [w649 _]
                tunnel: w616 -> [w648 w656]
                tunnel: w615 -> [w647 w654]
                tunnel: [w648 w662] -> w614
                tunnel: [w647 w661] -> w613
                frame False {
                }
                frame True {
                  # "Repete o ciclo de\nmovimento continuo."
                  n229 = call "Read window.vi"("error in (no error)"=w654, "Optics in"=w656) -> ("error out"=w653:errorcluster, "window"=w652:dbl, "Optics out"=w655:refnum<class "Optics.lvclass">)  [unwired: 7 in]
                  n230 = call "Read target.vi"("error in (no error)"=w653, "Optics in"=w655) -> ("error out"=w664:errorcluster, "target"=w660:dbl, "Optics out"=w663:refnum<class "Optics.lvclass">)  [unwired: 7 in]
                  n231 = call "Read position.vi"("error in (no error)"=w664, "Optics in"=w663) -> ("error out"=w661:errorcluster, "position"=w659:dbl, "Optics out"=w662:refnum<class "Optics.lvclass">)  [unwired: 7 in]
                  n232 = Subtract(x=w659, y=w660) -> (x-y=w658:dbl)
                  n233 = Absolute Value(x=w658) -> (abs(x)=w657:dbl)
                  n234 = Less Or Equal?(x=w657, y=w652) -> (x <= y?=→"on target 2":bool)
                }
              }
            }
          }
          n235 = call-dynamic "Write cmd.vi"("error in (no error)"=w582, "cmd"="", "Device in"=w583) -> ("error out"=w596:errorcluster, "Device out"=w597:refnum<class "Optics.lvclass">)  [unwired: 7 in]
        }
        frame 30 {
          # "S4ICS GMIR INIT NONE"
          # "WPROT/WPSEL/GFOC/GMIR/CALW/ASEL"
          # "comando INIT"
          n236 = call "Read name.vi"("error in (no error)"=w668, "Optics in"=w669) -> ("error out"=w667:errorcluster, "name"=w665:string, "Optics out"=w666:refnum<class "Optics.lvclass">)  [unwired: 7 in]
          n237 = Concatenate Strings(w665, " INIT NONE, " ("string")) -> (w673:string)
          n238 = call-dynamic "Write cmd.vi"("error in (no error)"=w667, "cmd"=w673, "Device in"=w666) -> ("error out"=w674:errorcluster, "Device out"=w675:refnum<class "Optics.lvclass">)  [unwired: 7 in]
          n239 = Increment(x=w671) -> (x+1=w672:i32)
        }
        frame 31 {
          # "60 x 1s = 1min de timeout para \nterminar o movimento do mecanismo"
          # "<name> <status> <position> <name_pos> <id_pos>"
          # "analisa resposta do ICS:    STATUS  esperando status=ACK"
          n240 = call-dynamic "Write Timer.vi"("error in (no error)"=w683, "Timer"=u32 60, "State Machine in"=w684) -> ("error out"=w682:errorcluster, "State Machine out"=w685:refnum<class "State Machine.lvclass">)  [unwired: 7 in]
          n241 = call-dynamic "Write State Machine.vi"("error in (no error)"=w682, "State Machine.lvclass"=w685, "Device in"=w686) -> ("error out"=w681:errorcluster, "Device out"=w680:refnum<class "Optics.lvclass">)  [unwired: 7 in]
          n242 = call "Read name.vi"("error in (no error)"=w681, "Optics in"=w680) -> ("error out"=w688:errorcluster, "name"=w687:string, "Optics out"=w689:refnum<class "Optics.lvclass">)  [unwired: 7 in]
          n243 = call-dynamic "Read resp.vi"("error in (no error)"=w688, "Device in"=w689) -> ("error out"=w694:errorcluster, "resp"=w699:string, "Device out"=w695:refnum<class "Optics.lvclass">)  [unwired: 7 in]
          n244 = Match Pattern(string=w699, regular expression=w687) -> (match substring=w697:string, after substring=w696:string)  [unwired: 1 in, 2 out]
          n245 = Equal?(x=w697, y=w687) -> (x = y?=w698:bool)
          n246 = case shown="False" w698 {
            tunnel: w696 -> [_ w713]
            tunnel: w695 -> [w702 w718]
            tunnel: w694 -> [w701 w717]
            tunnel: [w702 w728] -> w677
            tunnel: [w701 w727] -> w678
            tunnel: w693 -> [_ w723]
            tunnel: [0 w726] -> w692
            frame False {
            }
            frame True {
              # "retira \\s após o NOME"
              n247 = Match Pattern(string=w713, regular expression=" ") -> (after substring=w712:string)  [unwired: 1 in, 3 out]
              n248 = Match Pattern(string=w712, regular expression=" ") -> (before substring=w719:string, after substring=w716:string)  [unwired: 1 in, 2 out]
              n249 = call "Write mode.vi"("error in (no error)"=w717, "mode"=w719, "Optics in"=w718) -> ("error out"=w721:errorcluster, "Optics out"=w720:refnum<class "Optics.lvclass">)  [unwired: 7 in]
              n250 = Match Pattern(string=w716, regular expression=" ") -> (before substring=w725:string, after substring=w741:string)  [unwired: 1 in, 2 out]
              n251 = Match Pattern(string=w741, regular expression=" ") -> (before substring=w739:string, after substring=w738:string)  [unwired: 1 in, 2 out]
              n252 = call "Write condition.vi"("error in (no error)"=w721, "condition"=w725, "Optics in"=w720) -> ("error out"=w710:errorcluster, "Optics out"=w711:refnum<class "Optics.lvclass">)  [unwired: 7 in]
              n253 = Match Pattern(string=w738, regular expression=" ") -> (before substring=w737:string, after substring=w734:string)  [unwired: 1 in, 2 out]
              n254 = Fract/Exp String To Number(use system decimal point (T)=FALSE, string=w739) -> (number=w705:dbl)  [unwired: 2 in, 1 out]
              n255 = call "Read position.vi"("error in (no error)"=w710, "Optics in"=w711) -> ("error out"=w709:errorcluster, "position"=w704:dbl, "Optics out"=w708:refnum<class "Optics.lvclass">)  [unwired: 7 in]
              n256 = Not Equal?(x=w704, y=w705) -> (x != y?=w706:bool)
              n257 = Bundle By Name(cluster=w708, "Moving"=w706) -> (w707:refnum<class "Optics.lvclass">)
              n258 = call "Write position.vi"("error in (no error)"=w709, "position"=w705, "Optics in"=w707) -> ("error out"=w730:errorcluster, "Optics out"=w736:refnum<class "Optics.lvclass">)  [unwired: 7 in]
              n259 = Match Pattern(string=w734, regular expression=" ") -> (before substring=w733:string)  [unwired: 1 in, 3 out]
              n260 = Decimal String To Number(string=w733) -> (number=w732:i32)  [unwired: 2 in, 1 out]
              n261 = call "Write name_pos.vi"("error in (no error)"=w730, "name_pos"=w737, "Optics in"=w736) -> ("error out"=w729:errorcluster, "Optics out"=w731:refnum<class "Optics.lvclass">)  [unwired: 7 in]
              n262 = Equal?(x=w725, y="BUSY") -> (x = y?=w724:bool)
              n263 = call "Write id_pos.vi"("error in (no error)"=w729, "id_pos"=w732, "Optics in"=w731) -> ("error out"=w727:errorcluster, "Optics out"=w728:refnum<class "Optics.lvclass">)  [unwired: 7 in]
              n264 = case shown="True" w724 {
                tunnel: [w744 w745] -> w726
                tunnel: w723 -> [w744 w746]
                frame False {
                }
                frame True {
                  n265 = Increment(x=w746) -> (x+1=w745:i32)
                }
              }
            }
          }
          n266 = call-dynamic "Write cmd.vi"("error in (no error)"=w678, "cmd"="", "Device in"=w677) -> ("error out"=w690:errorcluster, "Device out"=w691:refnum<class "Optics.lvclass">)  [unwired: 7 in]
        }
        frame 32 {
          # "retira \\s após o NOME"
          # "<name> <status> <position> <name_pos> <id_pos>"
          # "analisa resposta do ICS:    STATUS  esperando status=READY"
          n267 = call "Verify Timer.vi"("error in (no error)"=w754, "State Machine in"=w756) -> ("error out"=w753:errorcluster, "timeout"=w752:bool, "State Machine out"=w755:refnum<class "State Machine.lvclass">)  [unwired: 7 in]
          n268 = call-dynamic "Write State Machine.vi"("error in (no error)"=w753, "State Machine.lvclass"=w755, "Device in"=w757) -> ("error out"=w750:errorcluster, "Device out"=w751:refnum<class "Optics.lvclass">)  [unwired: 7 in]
          n269 = call "Read name.vi"("error in (no error)"=w750, "Optics in"=w751) -> ("error out"=w762:errorcluster, "name"=w763:string, "Optics out"=w761:refnum<class "Optics.lvclass">)  [unwired: 7 in]
          n270 = call-dynamic "Read resp.vi"("error in (no error)"=w762, "Device in"=w761) -> ("error out"=w768:errorcluster, "resp"=w772:string, "Device out"=w769:refnum<class "Optics.lvclass">)  [unwired: 7 in]
          n271 = Match Pattern(string=w772, regular expression=w763) -> (match substring=w770:string, after substring=w760:string)  [unwired: 1 in, 2 out]
          n272 = Equal?(x=w770, y=w763) -> (x = y?=w771:bool)
          n273 = Match Pattern(string=w760, regular expression=" ") -> (after substring=w759:string)  [unwired: 1 in, 3 out]
          n274 = case shown="True" w771 {
            tunnel: w769 -> [w775 w796]
            tunnel: w768 -> [w774 w794]
            tunnel: [w775 w787] -> w748
            tunnel: [w774 w788] -> w749
            tunnel: w767 -> [_ w797]
            tunnel: [0 ("t") w800] -> w766
            tunnel: w759 -> [_ w789]
            tunnel: w752 -> [_ w776]
            frame False {
            }
            frame True {
              n275 = Match Pattern(string=w789, regular expression=" ") -> (before substring=w792:string, after substring=w791:string)  [unwired: 1 in, 2 out]
              n276 = Match Pattern(string=w791, regular expression=" ") -> (before substring=w799:string, after substring=w813:string)  [unwired: 1 in, 2 out]
              n277 = call "Write mode.vi"("error in (no error)"=w794, "mode"=w792, "Optics in"=w796) -> ("error out"=w793:errorcluster, "Optics out"=w795:refnum<class "Optics.lvclass">)  [unwired: 7 in]
              n278 = Match Pattern(string=w813, regular expression=" ") -> (before substring=w811:string, after substring=w810:string)  [unwired: 1 in, 2 out]
              n279 = call "Write condition.vi"("error in (no error)"=w793, "condition"=w799, "Optics in"=w795) -> ("error out"=w785:errorcluster, "Optics out"=w786:refnum<class "Optics.lvclass">)  [unwired: 7 in]
              n280 = Match Pattern(string=w810, regular expression=" ") -> (before substring=w809:string, after substring=w806:string)  [unwired: 1 in, 2 out]
              n281 = Fract/Exp String To Number(use system decimal point (T)=FALSE, string=w811) -> (number=w779:dbl)  [unwired: 2 in, 1 out]
              n282 = call "Read position.vi"("error in (no error)"=w785, "Optics in"=w786) -> ("error out"=w781:errorcluster, "position"=w780:dbl, "Optics out"=w784:refnum<class "Optics.lvclass">)  [unwired: 7 in]
              n283 = Not Equal?(x=w780, y=w779) -> (x != y?=w782:bool)
              n284 = Bundle By Name(cluster=w784, "Moving"=w782) -> (w783:refnum<class "Optics.lvclass">)
              n285 = call "Write position.vi"("error in (no error)"=w781, "position"=w779, "Optics in"=w783) -> ("error out"=w802:errorcluster, "Optics out"=w808:refnum<class "Optics.lvclass">)  [unwired: 7 in]
              n286 = Match Pattern(string=w806, regular expression=" ") -> (before substring=w805:string)  [unwired: 1 in, 3 out]
              n287 = Decimal String To Number(string=w805) -> (number=w804:i32)  [unwired: 2 in, 1 out]
              n288 = call "Write name_pos.vi"("error in (no error)"=w802, "name_pos"=w809, "Optics in"=w808) -> ("error out"=w801:errorcluster, "Optics out"=w803:refnum<class "Optics.lvclass">)  [unwired: 7 in]
              n289 = Not Equal?(x=w799, y="BUSY") -> (x != y?=w777:bool)
              n290 = call "Write id_pos.vi"("error in (no error)"=w801, "id_pos"=w804, "Optics in"=w803) -> ("error out"=w788:errorcluster, "Optics out"=w787:refnum<class "Optics.lvclass">)  [unwired: 7 in]
              n291 = case shown="False" w777 {
                tunnel: [w817 0 ("t")] -> w800
                tunnel: w797 -> [w818 _]
                tunnel: w776 -> [w816 _]
                frame False {
                  n292 = case shown="True" w816 {
                    tunnel: [w819 0 ("State")] -> w817
                    tunnel: w818 -> [w819 _]
                    frame False {
                    }
                    frame True {
                    }
                  }
                }
                frame True {
                }
              }
            }
          }
          n293 = call-dynamic "Write cmd.vi"("error in (no error)"=w749, "cmd"="", "Device in"=w748) -> ("error out"=w764:errorcluster, "Device out"=w765:refnum<class "Optics.lvclass">)  [unwired: 7 in]
        }
        frame 99 {
          # "WPROT/WPSEL/GFOC/GMIR/CALW/ASEL"
          n294 = call "Read name.vi"("error in (no error)"=w839, "Optics in"=w838) -> ("error out"=w833:errorcluster, "name"=w828:string, "Optics out"=w835:refnum<class "Optics.lvclass">)  [unwired: 7 in]
          n295 = call-dynamic "Read resp.vi"("error in (no error)"=w833, "Device in"=w835) -> ("error out"=w832:errorcluster, "resp"=w837:string, "Device out"=w834:refnum<class "Optics.lvclass">)  [unwired: 7 in]
          n296 = Match Pattern(string=w837, regular expression=w828) -> (match substring=w836:string, after substring=w829:string)  [unwired: 1 in, 2 out]
          n297 = Equal?(x=w836, y=w828) -> (x = y?=w831:bool)
          n298 = case shown="True" w831 {
            tunnel: w829 -> [_ w882]
            tunnel: w834 -> [w843 w866]
            tunnel: w832 -> [w844 w856]
            tunnel: [w843 w858] -> w827
            tunnel: [w844 w857] -> w826
            tunnel: [FALSE TRUE] -> w823
            frame False {
            }
            frame True {
              n299 = Match Pattern(string=w882, regular expression=" ") -> (after substring=w869:string)  [unwired: 1 in, 3 out]
              n300 = Match Pattern(string=w869, regular expression=" ") -> (before substring=w865:string, after substring=w864:string)  [unwired: 1 in, 2 out]
              n301 = call "Write mode.vi"("error in (no error)"=w856, "mode"=w865, "Optics in"=w866) -> ("error out"=w868:errorcluster, "Optics out"=w867:refnum<class "Optics.lvclass">)  [unwired: 7 in]
              n302 = Match Pattern(string=w864, regular expression=" ") -> (before substring=w859:string, after substring=w878:string)  [unwired: 1 in, 2 out]
              n303 = call "Write condition.vi"("error in (no error)"=w868, "condition"=w859, "Optics in"=w867) -> ("error out"=w853:errorcluster, "Optics out"=w854:refnum<class "Optics.lvclass">)  [unwired: 7 in]
              n304 = Match Pattern(string=w878, regular expression=" ") -> (before substring=w863:string, after substring=w875:string)  [unwired: 1 in, 2 out]
              n305 = call "Read position.vi"("error in (no error)"=w853, "Optics in"=w854) -> ("error out"=w852:errorcluster, "position"=w848:dbl, "Optics out"=w851:refnum<class "Optics.lvclass">)  [unwired: 7 in]
              n306 = Fract/Exp String To Number(use system decimal point (T)=FALSE, string=w863) -> (number=w849:dbl)  [unwired: 2 in, 1 out]
              n307 = Not Equal?(x=w848, y=w849) -> (x != y?=w847:bool)
              n308 = Bundle By Name(cluster=w851, "Moving"=w847) -> (w850:refnum<class "Optics.lvclass">)
              n309 = Match Pattern(string=w875, regular expression=" ") -> (before substring=w846:string, after substring=w861:string)  [unwired: 1 in, 2 out]
              n310 = call "Write position.vi"("error in (no error)"=w852, "position"=w849, "Optics in"=w850) -> ("error out"=w872:errorcluster, "Optics out"=w877:refnum<class "Optics.lvclass">)  [unwired: 7 in]
              n311 = Match Pattern(string=w861, regular expression=" ") -> (after substring=w860:string)  [unwired: 1 in, 3 out]
              n312 = call "Write name_pos.vi"("error in (no error)"=w872, "name_pos"=w846, "Optics in"=w877) -> ("error out"=w871:errorcluster, "Optics out"=w873:refnum<class "Optics.lvclass">)  [unwired: 7 in]
              n313 = Decimal String To Number(string=w860) -> (number=w874:i32)  [unwired: 2 in, 1 out]
              n314 = call "Write id_pos.vi"("error in (no error)"=w871, "id_pos"=w874, "Optics in"=w873) -> ("error out"=w857:errorcluster, "Optics out"=w858:refnum<class "Optics.lvclass">)  [unwired: 7 in]
            }
          }
          n315 = call "Write connected.vi"("error in (no error)"=w826, "connected"=w823, "Device in"=w827) -> ("error out"=w824:errorcluster, "Device out"=w825:refnum<class "Optics.lvclass">)  [unwired: 7 in]
          n316 = call-dynamic "Write cmd.vi"("error in (no error)"=w824, "cmd"="", "Device in"=w825) -> ("error out"=w840:errorcluster, "Device out"=w841:refnum<class "Optics.lvclass">)  [unwired: 7 in]
        }
      }
      n317 = call-dynamic "Read State Machine.vi"("error in (no error)"=w11, "Device in"=w18) -> ("error out"=w14:errorcluster, "State Machine.lvclass"=w17:refnum<class "State Machine.lvclass">, "Device out"=w16:refnum<class "Optics.lvclass">)  [unwired: 7 in]
      n318 = call "Next State.vi"("error in (no error)"=w14, "New_State"=w12, "State Machine in"=w17) -> ("error out"=w13:errorcluster, "State Machine out"=w19:refnum<class "State Machine.lvclass">)  [unwired: 7 in]
      n319 = call-dynamic "Write State Machine.vi"("error in (no error)"=w13, "State Machine.lvclass"=w19, "Device in"=w16) -> ("error out"=w10:errorcluster, "Device out"=w15:refnum<class "Optics.lvclass">)  [unwired: 7 in]
    }
    frame Error {
    }
  }
  "error out" <- w1
  "Optics out" <- w2
